vi "HandleClients.vi"(8 "error in (no error)":errorcluster, 11 "GuiderSetup in":refnum<class "GuiderSetup.lvclass">) -> (0 "error out":errorcluster, 3 "GuiderSetup out":refnum<class "GuiderSetup.lvclass">)   [LabVIEW 2018, in "GuiderSetup.lvclass"]
uses:
  GuiderSetup.lvclass
  GuiderSetup.lvclass/GuiderSetup.ctl
  PublisherGS/PublisherGS.lvclass
  AG/AG.lvclass
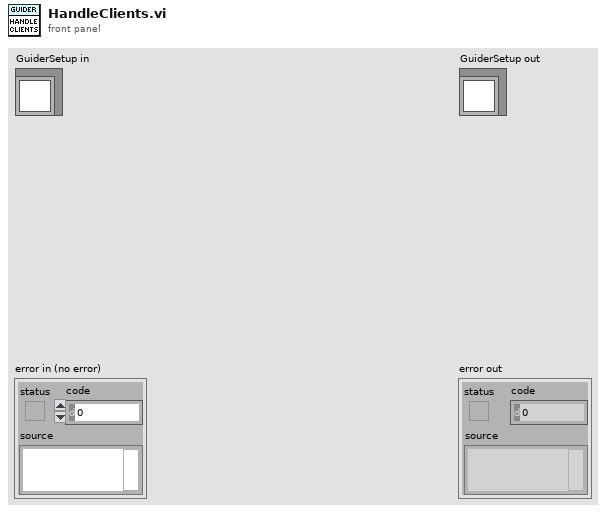
[diagram p1: front panel]
types:
  T1 = cluster{"FocusPhot":dbl, "FocusPolar":dbl, "FocusEffic":dbl, "FocusInstrum":dbl, "ICS":bool, "AG":bool, "broker":string, "timestamp":string}
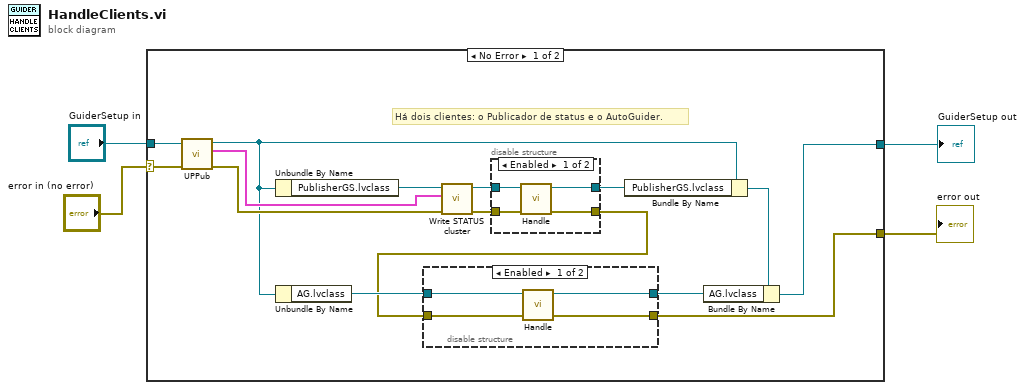
[diagram p0: block diagram]
diagram:
  n1 = case shown="No Error" "error in (no error)" {
    selector: "error in (no error)" -> [w18 w32]
    tunnel: "GuiderSetup in" -> [w19 w33]
    tunnel: [w5 w33] -> w2
    tunnel: [w8 w32] -> w1
    frame No Error {
      # "Há dois clientes: o Publicador de status e o AutoGuider."
      n2 = call-dynamic "UPPub.vi"("error in (no error)"=w18, "GuiderSetup in"=w19) -> ("error out"=w14:errorcluster, "STATUS cluster"=w15:T1, "GuiderSetup out"=w6:refnum<class "GuiderSetup.lvclass">)  [unwired: 7 in]
      n3 = Unbundle By Name(w6) -> ("PublisherGS.lvclass"=w17:refnum<class "PublisherGS.lvclass">)
      n4 = Unbundle By Name(w6) -> ("AG.lvclass"=w11:refnum<class "AG.lvclass">)
      n5 = call-dynamic "Write STATUS cluster.vi"("error in (no error)"=w14, "STATUS cluster"=w15, "PublisherGS in"=w17) -> ("error out"=w13:errorcluster, "PublisherGS out"=w16:refnum<class "PublisherGS.lvclass">)  [unwired: 7 in]
      n6 = disable-structure shown="Enabled" {
        disable-tunnel: w16 -> [w23 w25]
        disable-tunnel: w13 -> [w22 w24]
        disable-tunnel: [w21 w25] -> w12
        disable-tunnel: [w20 w24] -> w9
        frame Enabled {
          n7 = call-dynamic "Handle.vi"("error in (no error)"=w22, "PublisherGS in"=w23) -> ("error out"=w20:errorcluster, "PublisherGS out"=w21:refnum<class "PublisherGS.lvclass">)  [unwired: 8 in]
        }
        frame Disabled {
        }
      }
      n8 = disable-structure shown="Enabled" {
        disable-tunnel: w11 -> [w29 w31]
        disable-tunnel: [w28 w31] -> w10
        disable-tunnel: w9 -> [w27 w30]
        disable-tunnel: [w26 w30] -> w8
        frame Enabled {
          n9 = call-dynamic "Handle.vi"("error in (no error)"=w27, "AG in"=w29) -> ("error out"=w26:errorcluster, "AG out"=w28:refnum<class "AG.lvclass">)  [unwired: 8 in]
        }
        frame Disabled {
        }
      }
      n10 = Bundle By Name(cluster=w6, "PublisherGS.lvclass"=w12) -> (w7:refnum<class "GuiderSetup.lvclass">)
      n11 = Bundle By Name(cluster=w7, "AG.lvclass"=w10) -> (w5:refnum<class "GuiderSetup.lvclass">)
    }
    frame Error {
    }
  }
  "error out" <- w1
  "GuiderSetup out" <- w2
